vi "tdms.vi"() -> ()   [LabVIEW 2020]
uses:
  <vilib>/Waveform/WDTFileIO.llb/Read Waveform from File.vi
  <vilib>/measure/NI_MABase.lvlib
panel:
  out "Waveform Graph 2":waveform(dbl)(graph)
  out "Waveform Graph":waveform(dbl)(graph)
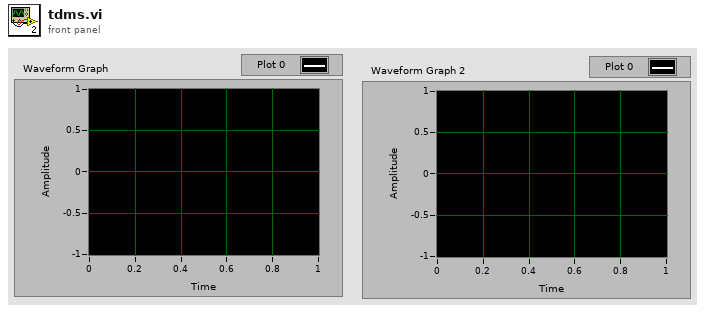
[diagram p1: front panel]
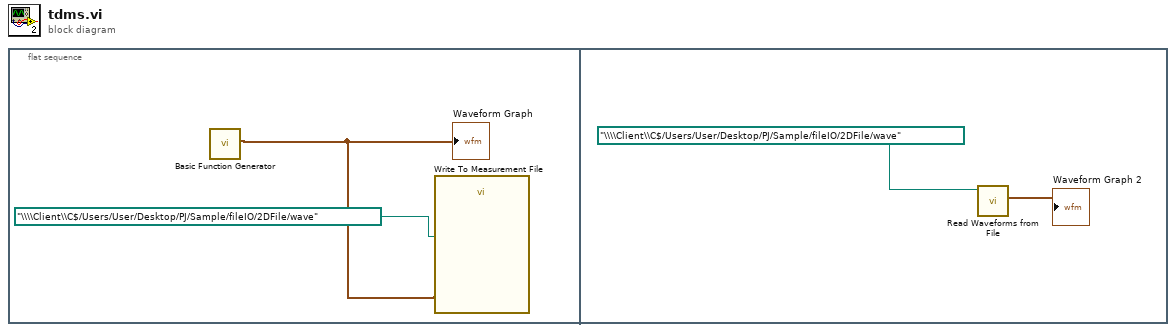
[diagram p0: block diagram]
diagram:
  n1 = flat-sequence {
    frame #0 {
      n2 = call <vilib>:"Basic Function Generator.vi"() -> ("signal out"=w1:waveform(dbl))  [unwired: 9 in, 2 out]
      "Waveform Graph" <- w1
      n3 = call "Write To Measurement File"("Signals"=w1, "Filename"=path "\\\\Client\\C$/Users/User/Desktop/PJ/Sample/fileIO/2DFile/wave" ("file path (dialog if empty)")) -> ()  [unwired: 15 in, 3 out]
    }
    frame #1 {
      n4 = call-poly <vilib>:"Read Waveforms from File.vi"("file path (dialog if empty)"=path "\\\\Client\\C$/Users/User/Desktop/PJ/Sample/fileIO/2DFile/wave") -> ("first waveform in record"=→"Waveform Graph 2":waveform(dbl))  [unwired: 5 in, 3 out]
    }
  }
